vi "Get Meta Data.vi"(0 "Measurement Client Wrapper in":refnum<class "Measurement Client Wrapper.lvclass">, 11 "error in":errorcluster) -> (4 "Measurement Client Wrapper out":refnum<class "Measurement Client Wrapper.lvclass">, 15 "error out":errorcluster)   [LabVIEW 2020, in "Measurement Client Wrapper.lvclass"]
uses:
  Measurement Client Wrapper.lvclass
  Typedefs/Measurement Parameters.ctl
  Typedefs/MeasurementConfigurationParameters.ctl
  <vilib>/TAF/LabVIEW Measurement Client/RPC Messages/ni_measurements_v1_Type.ctl
  Typedefs/MeasurementOutputParameters.ctl
  <vilib>/TAF/LabVIEW Measurement Client/RPC Messages/google_protobuf_Any.ctl
  Measurement Client Wrapper.lvclass/Measurement Client Wrapper.ctl
  <vilib>/TAF/LabVIEW Measurement Client/Measurement_client-release.lvlib
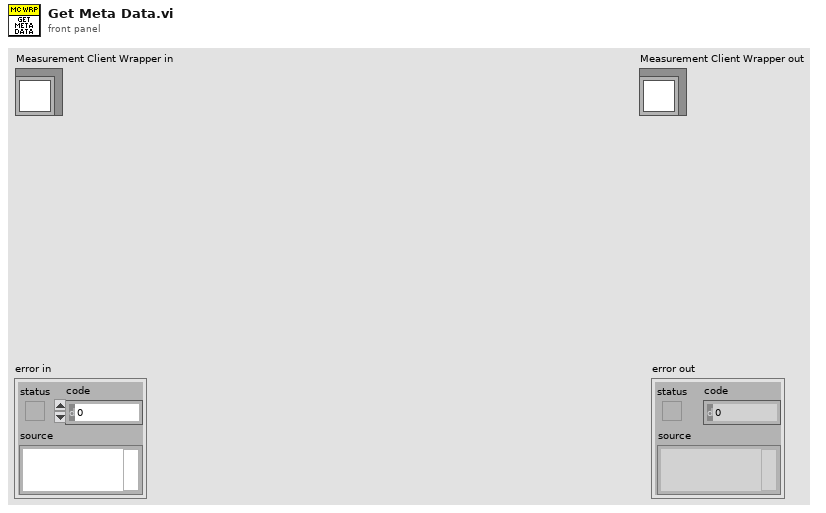
[diagram p1: front panel]
types:
  T1 = typedef "Measurement Client Wrapper.lvclass/Measurement Parameters.ctl" = cluster{"Configuration Parameters MessageType":string, "Configuration Parameter[]":T2[], "Output Parameters MessageType":string, "Output Parameter[]":T4[], "google_protobuf_Any":T5}
  T2 = typedef "Measurement Client Wrapper.lvclass/MeasurementConfigurationParameters.ctl" = cluster{"protobuf_id":u32, "type":T3, "name":string, "repeated":bool}
  T3 = typedef "Measurement_client-release.lvlib/ni_measurements_v1_Type.ctl" = enum32{"TYPE_UNSPECIFIED", "TYPE_DOUBLE", "TYPE_FLOAT", "TYPE_INT64", "TYPE_UINT64", "TYPE_INT32", "TYPE_FIXED64", "TYPE_FIXED32", "TYPE_BOOL", "TYPE_STRING", "TYPE_GROUP", "TYPE_MESSAGE", "TYPE_BYTES", "TYPE_UINT32", "TYPE_ENUM", "TYPE_SFIXED32", "TYPE_SFIXED64", "TYPE_SINT32", "TYPE_SINT64"}
  T4 = typedef "Measurement Client Wrapper.lvclass/MeasurementOutputParameters.ctl" = cluster{"protobuf_id":u32, "type":T3, "name":string, "repeated":bool}
  T5 = typedef "Measurement_client-release.lvlib/google_protobuf_Any.ctl" = cluster{"type_url":string, "value":u8[]}
  T6 = typedef "gprc-lvsupport-release.lvlib/grpcId.ctl" = u64
  T7 = typedef "Measurement_client-release.lvlib/ni_measurements_v1_GetMetadataResponse.ctl" = cluster{"measurement_details":T8, "measurement_parameters":T9, "user_interface_details":T12}
  T8 = typedef "Measurement_client-release.lvlib/ni_measurements_v1_MeasurementDetails.ctl" = cluster{"display_name":string, "version":string, "measurement_type":string, "product_type":string}
  T9 = typedef "Measurement_client-release.lvlib/ni_measurements_v1_MeasurementParameters.ctl" = cluster{"configuration_parameters_messagetype":string, "configuration_parameters":T10[], "configuration_defaults":T5, "outputs_message_type":string, "outputs":T11[]}
  T10 = typedef "Measurement_client-release.lvlib/ni_measurements_v1_ConfigurationParameter.ctl" = cluster{"protobuf_id":u32, "type":i32, "name":string, "repeated":bool}
  T11 = typedef "Measurement_client-release.lvlib/ni_measurements_v1_Output.ctl" = cluster{"protobuf_id":u32, "type":i32, "name":string, "repeated":bool}
  T12 = typedef "Measurement_client-release.lvlib/ni_measurements_v1_UserInterfaceDetails.ctl" = cluster{"configuration_ui_url":string}
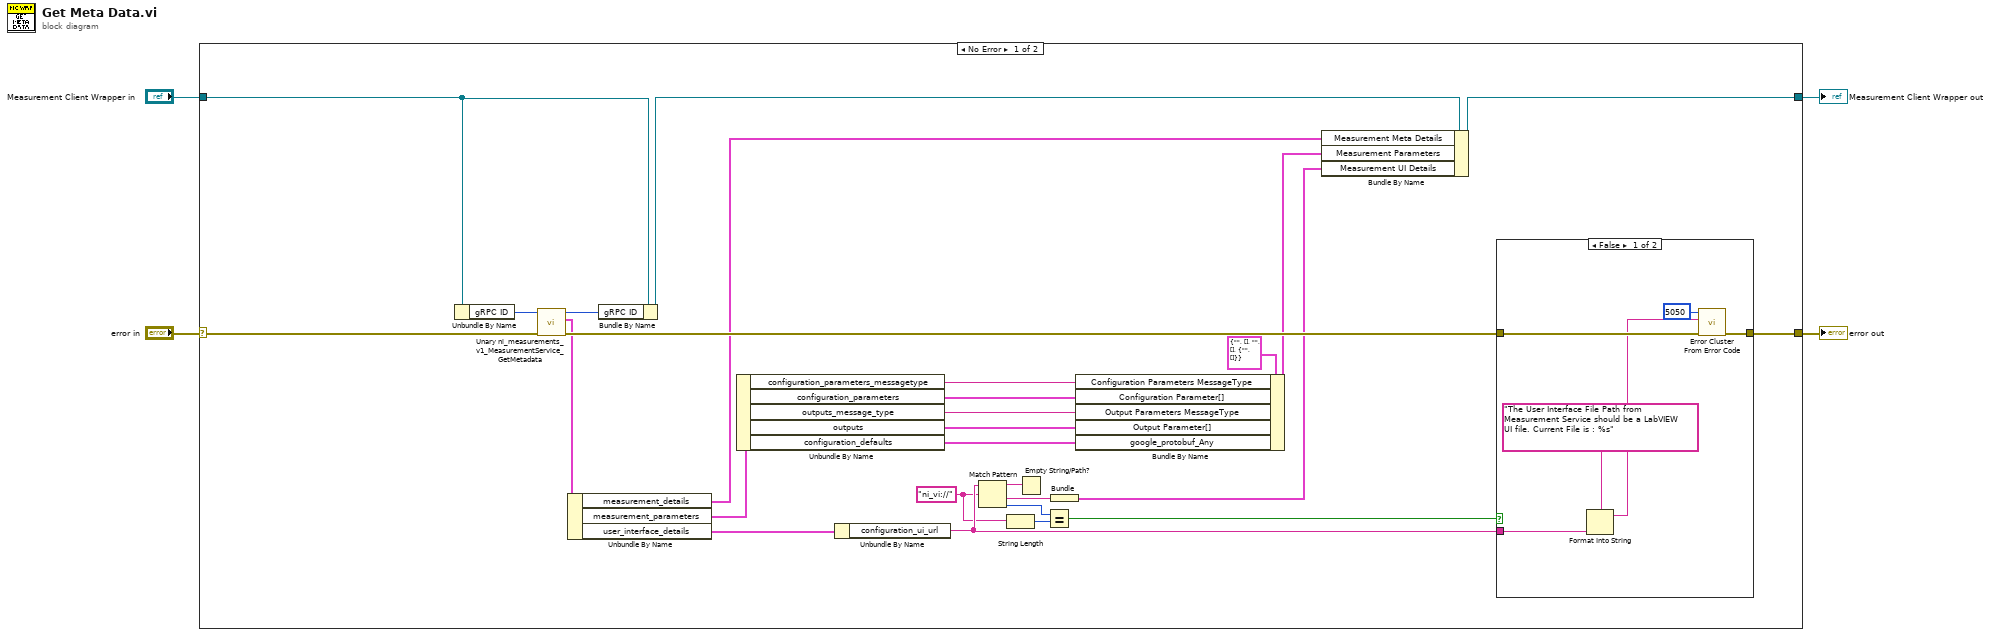
[diagram p0: block diagram]
diagram:
  n1 = case shown="No Error" "error in" {
    selector: "error in" -> [w31 w40]
    tunnel: [w12 w40] -> w3
    tunnel: [w30 w39] -> w1
    tunnel: "Measurement Client Wrapper in" -> [w28 w39]
    frame No Error {
      w7 = "ni_vi://" ("regular expression")
      n2 = Unbundle By Name(w28) -> ("gRPC ID"=w27:T6)
      n3 = call <vilib>:"Unary ni_measurements_v1_MeasurementService_GetMetadata.vi"("error in"=w31, "gRPC ID"=w27) -> ("error out"=w29:errorcluster, "Response Data"=w25:T7, "gRPC ID out"=w26:T6)  [unwired: 7 in]
      n4 = Unbundle By Name(w25) -> ("measurement_details"=w19:T8, "measurement_parameters"=w24:T9, "user_interface_details"=w15:T12)
      n5 = Bundle By Name(cluster=w28, "gRPC ID"=w26) -> (w20:refnum<class "Measurement Client Wrapper.lvclass">)
      n6 = Unbundle By Name(w24) -> ("configuration_parameters_messagetype"=w21:string, "configuration_parameters"=w17:T10[], "outputs_message_type"=w22:string, "outputs"=w16:T11[], "configuration_defaults"=w5:T5)
      n7 = Unbundle By Name(w15) -> ("configuration_ui_url"=w11:string)
      n8 = Match Pattern(string=w11, regular expression=w7) -> (before substring=w10:string, after substring=w14:string, offset past match=w9:i32)  [unwired: 1 in, 1 out]
      n9 = String Length(string=w7) -> (length=w8:i32)
      n10 = Empty String/Path?(string/path=w10) -> ()  [unwired: 1 out]
      n11 = Equal?(x=w9, y=w8) -> (x = y?=w6:bool)
      n12 = Bundle("configuration_ui_url"=w14) -> (w13:cluster{"configuration_ui_url":string})  [unwired: 1 in]
      n13 = Bundle By Name(cluster=T1 {"Configuration Parameters MessageType"="", "Configuration Parameter[]"=[], "Output Parameters MessageType"="", "Output Parameter[]"=[], "google_protobuf_Any"={"type_url"="", "value"=[]}} ("Measurement Parameters"), "Configuration Parameters MessageType"=w21, "Configuration Parameter[]"=w17, "Output Parameters MessageType"=w22, "Output Parameter[]"=w16, "google_protobuf_Any"=w5) -> (w18:T1)
      n14 = Bundle By Name(cluster=w20, "Measurement Meta Details"=w19, "Measurement Parameters"=w18, "Measurement UI Details"=w13) -> (w30:refnum<class "Measurement Client Wrapper.lvclass">)
      n15 = case shown="False" w6 {
        tunnel: w29 -> [w37 w38]
        tunnel: [w36 w38] -> w12
        tunnel: w11 -> [w33 _]
        frame False {
          n16 = Format Into String(format string="The User Interface File Path from Measurement Service should be a LabVIEW UI file. Current File is : %s" ("error message (\"\")"), w33) -> (resulting string=w32:string)  [unwired: 2 in, 1 out]
          n17 = call <vilib>:"Error Cluster From Error Code.vi"("error in (no error)"=w37, "error message (\"\")"=w32, "error code (0)"=5050) -> ("error out"=w36:errorcluster)  [unwired: 6 in]
        }
        frame True {
        }
      }
    }
    frame Error {
    }
  }
  "error out" <- w3
  "Measurement Client Wrapper out" <- w1
